vi "Initializing.vi"(11 "Needs Init?":T1) -> (2 "Go to Idling":T1, 3 "Retry Initialization":T1)   [LabVIEW 2017]
uses:
  <extravilib>/ChannelInstances/Messenger-bool/))Channel.ctl
  <extravilib>/ChannelInstances/Messenger-bool/Read With Abort.vi
  <extravilib>/ChannelInstances/Messenger-bool/Write With Abort.vi
  <resource>/Channels/Messenger/Read With Abort.vi
  <vilib>/ChannelSupport/Channel Message/Read ID.vi
  <resource>/Channels/Messenger/Write With Abort.vi
  <extravilib>/ChannelInstances/Messenger-bool/Wrapper.lvclass
  C:/Program Files (x86)/National Instruments/LabVIEW 2017/vi.lib/ChannelSupport/Channel Message/Channel Message.lvclass
  <resource>/Channels/Messenger/Endpoint.vi
  <extravilib>/ChannelInstances/Messenger-bool/Unwrap.vi
  <extravilib>/ChannelInstances/Messenger-bool/Wrap.vi
  <extravilib>/ChannelInstances/Messenger-bool.lvlib
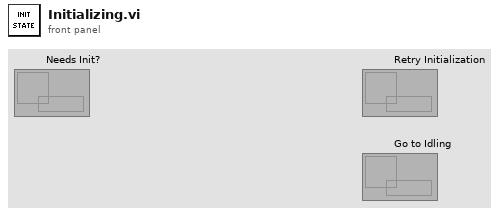
[diagram p1: front panel]
types:
  T1 = typedef "Messenger-bool.lvlib/))Channel.ctl" = refnum<queue>
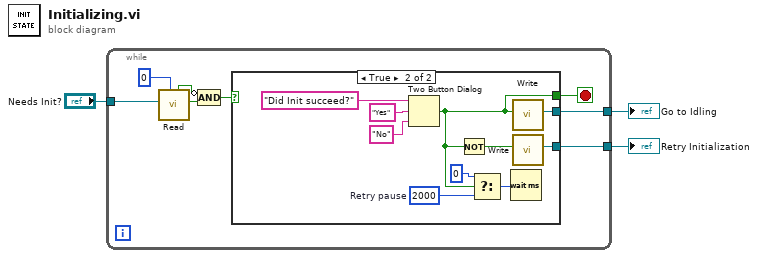
[diagram p0: block diagram]
diagram:
  n1 = while {
    tunnel: "Needs Init?" -> [w11]
    tunnel: [w10] -> w2
    tunnel: [w9] -> w1
    stop <- w4 stop-if-true
    n2 = call <extravilib>:"Read.vi"("timeout in ms (-1)"=0, "channel"=w11) -> ("element"=w6:bool, "timedout?"=w7:bool)  [unwired: 6 in, 2 out]
    n3 = Compound Arithmetic op=AND(invert w7, w6) -> (w5:bool)
    n4 = case shown="True" w5 {
      tunnel: [_ w17] -> w10
      tunnel: [_ w16] -> w9
      tunnel: [_ w14] -> w4
      frame False {
      }
      frame True {
        w12 = u32 2000  # Retry pause
        n5 = Two Button Dialog(message="Did Init succeed?", 1:"No" ("F button name (\"Cancel\")"), 2:"Yes" ("T button name (\"OK\")")) -> (T button?=w14:bool)
        n6 = Not(x=w14) -> (.not. x?=w18:bool)
        n7 = Select(t=u32 0, s=w14, f=w12) -> (s? t:f=w15:u32)
        n8 = Wait (ms)(milliseconds to wait=w15) -> ()  [unwired: 1 out]
        n9 = call <extravilib>:"Write.vi"("element"=w14) -> ("channel"=w16:T1)  [unwired: 8 in, 2 out]
        n10 = call <extravilib>:"Write.vi"("element"=w18) -> ("channel"=w17:T1)  [unwired: 8 in, 2 out]
      }
    }
  }
  "Retry Initialization" <- w2
  "Go to Idling" <- w1
